vi "OAT Output Buffered Data (XY, 1 Chan).vi"(0 "XY signal":cluster{"X":dbl[], "Y":dbl[]} {"X" format="%.2f"; "Y" format="%.2f"}, 2 "reset? (F)":bool, 7 "position info":T1, 11 "error in (no error)":errorcluster, 12 "buffer settings":T2) -> (4 "buffered XY signal":cluster{"X":dbl[], "Y":dbl[]} {"X" format="%.2f"; "Y" format="%.2f"}, 8 "buffered position info":T1, 15 "error out":errorcluster)   [LabVIEW 2017, in "SoundVib_OAUtility.lvlib"]
doc: "Buffers the input signals and returns them in first-in first-out (FIFO) mode. Use <B>buffer settings</B> to set the buffer size and units. Each instance of this VI maintains its own state; use the N Waveforms instance of this VI to process an array of channels. Wire data to the <B>XY signal</B> input to determine the polymorphic instance to use or manually select the instance."
uses:
  <vilib>/addons/Sound and Vibration/Order Analysis/Utility/SoundVib_OAUtility.lvlib
  <vilib>/addons/Sound and Vibration/Order Analysis/Utility/SubVIs/oa_Buffer Settings.ctl
  <vilib>/addons/Sound and Vibration/Order Analysis/Misc/OAT Position Info.ctl
  <vilib>/addons/_NISVFA/_Shared subVIs/Common/svc_Get Array Subset (Index).vi
  <vilib>/addons/_NISVFA/_Shared subVIs/Common/svc_Coerce Index and Length.vi
  <vilib>/addons/_NISVFA/_Shared subVIs/Common/svc_Conditional Merge Error.vi
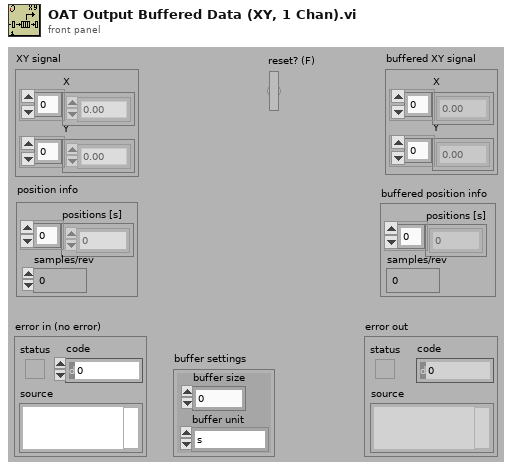
[diagram p1: front panel]
types:
  T1 = typedef "OAT Position Info.ctl" = cluster{"positions [s]":dbl[], "samples/rev":dbl}
  T2 = typedef "SoundVib_OAUtility.lvlib/oa_Buffer Settings.ctl" = cluster{"buffer size":dbl, "buffer unit":enum16{"s", "revolution", "# of samples"}}
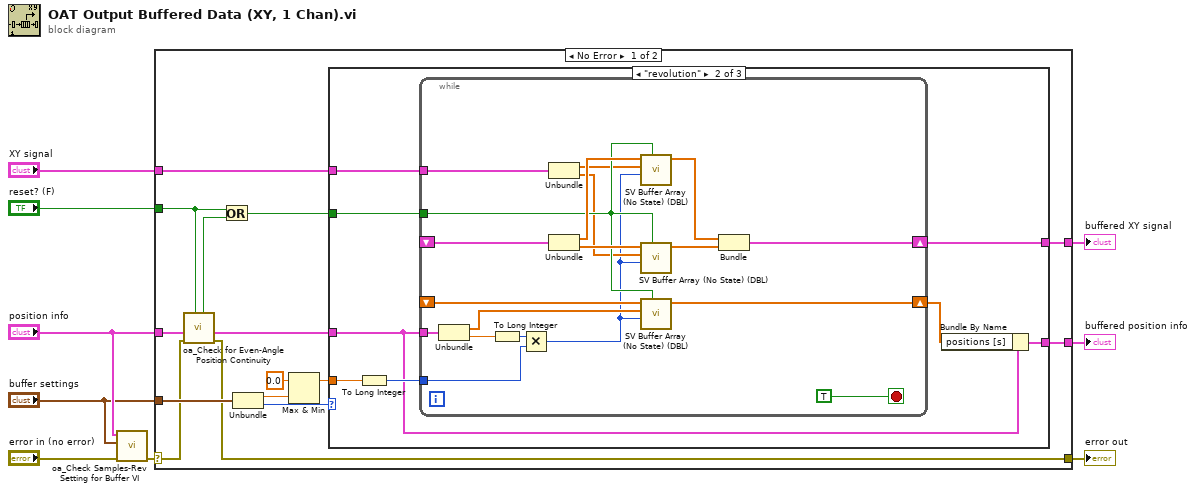
[diagram p0: block diagram]
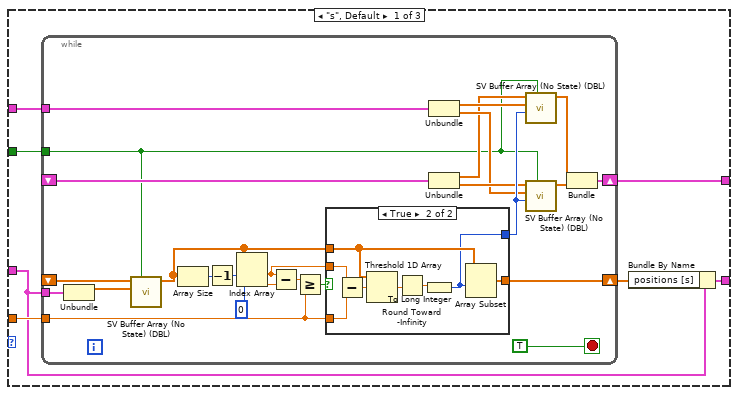
[diagram p2: hidden frame]
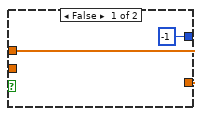
[diagram p3: hidden frame]
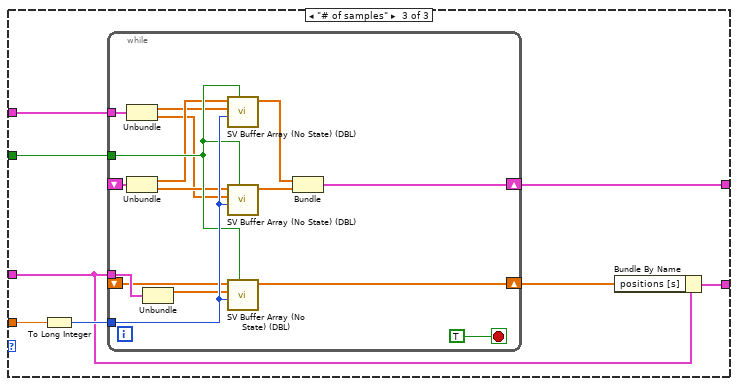
[diagram p4: hidden frame]
diagram:
  n1 = call <vilib>:"oa_Check Samples-Rev Setting for Buffer VI.vi"("error in (no error)"="error in (no error)", "buffer settings"="buffer settings", "position info"="position info") -> ("error out"=w5:errorcluster)  [unwired: 8 in]
  n2 = case shown="No Error" w5 {
    selector: w5 -> [w16 w118]
    tunnel: [w15 w118] -> w9
    tunnel: "buffer settings" -> [w24 _]
    tunnel: "XY signal" -> [w21 _]
    tunnel: "reset? (F)" -> [w14 _]
    tunnel: [w20 _] -> w6
    tunnel: "position info" -> [w17 _]
    tunnel: [w10 _] -> w1
    frame No Error {
      n3 = call <vilib>:"oa_Check for Even-Angle Position Continuity.vi"("reset in"=w14, "error in (no error)"=w16, "even-angle position info"=w17) -> ("error out"=w15:errorcluster, "even-angle position info dup"=w11:T1, "position not continuous"=w12:bool)  [unwired: 6 in]
      n4 = Or(x=w14, y=w12) -> (x .or. y?=w13:bool)
      n5 = Unbundle(w24) -> ("buffer size"=w18:dbl, "buffer unit"=w19:enum16{"s", "revolution", "# of samples"})
      n6 = Max & Min(x=0.0, y=w18) -> (max(x,y)=w22:dbl)  [unwired: 1 out]
      n7 = case shown="\"revolution\"" w19 {
        tunnel: w22 -> [w31 w72 w98]
        tunnel: w21 -> [w30 w74 w101]
        tunnel: w13 -> [w29 w73 w100]
        tunnel: [w28 w70 w99] -> w20
        tunnel: w11 -> [w27 w67 w95]
        tunnel: [w25 w69 w94] -> w10
        frame "s", Default {
          n8 = while {
            tunnel: w31 -> [w48]
            tunnel: w30 -> [w46]
            shift-right: [w43] -> w28
            shift-left: _ -> [w47]
            tunnel: w29 -> [w32]
            shift-right: [w45] -> w26
            shift-left: _ -> [w34]
            tunnel: w27 -> [w44]
            stop <- TRUE stop-if-true
            n9 = Unbundle(w44) -> ("positions [s]"=w35:dbl[])  [unwired: 1 out]
            n10 = call <vilib>:"SV Buffer Array (No State) (DBL).vi"("clear buffer (False)"=w32, "Y"=w35, "buffer in"=w34) -> ("buffer out"=w33:dbl[])  [unwired: 8 in]
            n11 = Array Size(array=w33) -> (size(s)=w56:i32)
            n12 = Decrement(x=w56) -> (x-1=w55:i32)
            n13 = Index Array(array=w33, index #1=w55, index #2=0 ("index")) -> (element #1=w49:dbl, element #2=w53:dbl)
            n14 = Subtract(x=w49, y=w53) -> (x-y=w52:dbl)
            n15 = Greater Or Equal?(x=w52, y=w48) -> (x >= y?=w51:bool)
            n16 = case shown="True" w51 {
              tunnel: w33 -> [w58 w63]
              tunnel: w49 -> [_ w66]
              tunnel: w48 -> [_ w65]
              tunnel: [w58 w62] -> w45
              tunnel: [-1 w59] -> w42
              frame False {
              }
              frame True {
                n17 = Subtract(x=w66, y=w65) -> (x-y=w64:dbl)
                n18 = Threshold 1D Array(2:w64, 3:w63) -> (0:w61:dbl)  [unwired: 1 in]
                n19 = Round Toward -Infinity(1:w61) -> (0:w60:dbl)
                n20 = To Long Integer(number=w60) -> (32bit integer=w59:i32)
                n21 = Array Subset(array=w63, index=w59) -> (w62:dbl[])  [unwired: 1 in]
              }
            }
            n22 = Unbundle(w46) -> ("X"=w37:dbl[], "Y"=w38:dbl[])
            n23 = Unbundle(w47) -> ("buffer out"=w36:dbl[], "buffer out"=w39:dbl[])
            n24 = call <vilib>:"SV Buffer Array (No State) (DBL).vi"("clear buffer (False)"=w32, "buffer length  [samples] (-1 = unlimited)"=w42, "Y"=w37, "buffer in"=w36) -> ("buffer out"=w41:dbl[])  [unwired: 7 in]
            n25 = call <vilib>:"SV Buffer Array (No State) (DBL).vi"("clear buffer (False)"=w32, "buffer length  [samples] (-1 = unlimited)"=w42, "Y"=w38, "buffer in"=w39) -> ("buffer out"=w40:dbl[])  [unwired: 7 in]
            n26 = Bundle("buffer out"=w41, "buffer out"=w40) -> (w43:cluster{"buffer out":dbl[], "buffer out":dbl[]})  [unwired: 1 in]
          }
          n27 = Bundle By Name(cluster=w27, "positions [s]"=w26) -> (w25:T1)
        }
        frame "revolution" {
          n28 = To Long Integer(number=w72) -> (32bit integer=w71:i32)
          n29 = while {
            tunnel: w74 -> [w93]
            shift-right: [w91] -> w70
            shift-left: _ -> [w90]
            tunnel: w73 -> [w79]
            tunnel: w71 -> [w88]
            tunnel: w67 -> [w87]
            shift-right: [w85] -> w68
            shift-left: _ -> [w80]
            stop <- TRUE stop-if-true
            n30 = Unbundle(w87) -> ("positions [s]"=w76:dbl[], "samples/rev"=w86:dbl)
            n31 = To Long Integer(number=w86) -> (32bit integer=w89:i32)
            n32 = Multiply(x=w89, y=w88) -> (x*y=w75:i32)
            n33 = Unbundle(w93) -> ("X"=w78:dbl[], "Y"=w77:dbl[])
            n34 = Unbundle(w90) -> ("buffer out"=w82:dbl[], "buffer out"=w81:dbl[])
            n35 = call <vilib>:"SV Buffer Array (No State) (DBL).vi"("clear buffer (False)"=w79, "buffer length  [samples] (-1 = unlimited)"=w75, "Y"=w78, "buffer in"=w82) -> ("buffer out"=w83:dbl[])  [unwired: 7 in]
            n36 = call <vilib>:"SV Buffer Array (No State) (DBL).vi"("clear buffer (False)"=w79, "buffer length  [samples] (-1 = unlimited)"=w75, "Y"=w77, "buffer in"=w81) -> ("buffer out"=w84:dbl[])  [unwired: 7 in]
            n37 = call <vilib>:"SV Buffer Array (No State) (DBL).vi"("clear buffer (False)"=w79, "buffer length  [samples] (-1 = unlimited)"=w75, "Y"=w76, "buffer in"=w80) -> ("buffer out"=w85:dbl[])  [unwired: 7 in]
            n38 = Bundle("buffer out"=w83, "buffer out"=w84) -> (w91:cluster{"buffer out":dbl[], "buffer out":dbl[]})  [unwired: 1 in]
          }
          n39 = Bundle By Name(cluster=w67, "positions [s]"=w68) -> (w69:T1)
        }
        frame "# of samples" {
          n40 = To Long Integer(number=w98) -> (32bit integer=w97:i32)
          n41 = while {
            tunnel: w101 -> [w117]
            shift-right: [w115] -> w99
            shift-left: _ -> [w114]
            tunnel: w100 -> [w109]
            tunnel: w97 -> [w110]
            tunnel: w95 -> [w113]
            shift-right: [w108] -> w96
            shift-left: _ -> [w102]
            stop <- TRUE stop-if-true
            n42 = Unbundle(w117) -> ("X"=w103:dbl[], "Y"=w104:dbl[])
            n43 = Unbundle(w114) -> ("buffer out"=w105:dbl[], "buffer out"=w106:dbl[])
            n44 = Unbundle(w113) -> ("positions [s]"=w107:dbl[])  [unwired: 1 out]
            n45 = call <vilib>:"SV Buffer Array (No State) (DBL).vi"("clear buffer (False)"=w109, "buffer length  [samples] (-1 = unlimited)"=w110, "Y"=w103, "buffer in"=w105) -> ("buffer out"=w112:dbl[])  [unwired: 7 in]
            n46 = call <vilib>:"SV Buffer Array (No State) (DBL).vi"("clear buffer (False)"=w109, "buffer length  [samples] (-1 = unlimited)"=w110, "Y"=w104, "buffer in"=w106) -> ("buffer out"=w111:dbl[])  [unwired: 7 in]
            n47 = call <vilib>:"SV Buffer Array (No State) (DBL).vi"("clear buffer (False)"=w109, "buffer length  [samples] (-1 = unlimited)"=w110, "Y"=w107, "buffer in"=w102) -> ("buffer out"=w108:dbl[])  [unwired: 7 in]
            n48 = Bundle("buffer out"=w112, "buffer out"=w111) -> (w115:cluster{"buffer out":dbl[], "buffer out":dbl[]})  [unwired: 1 in]
          }
          n49 = Bundle By Name(cluster=w95, "positions [s]"=w96) -> (w94:T1)
        }
      }
    }
    frame Error {
    }
  }
  "error out" <- w9
  "buffered XY signal" <- w6
  "buffered position info" <- w1
